vi "Get Position.vi"(8 "error in (no error)":errorcluster, 11 "KUKA youBot gripper motor_EtherCAT in":refnum<class "NI_Robotics_KUKA youBot Gripper Motor_EtherCAT.lvclass">) -> (0 "error out":errorcluster, 2 "position (m)":dbl, 3 "KUKA youBot gripper motor_EtherCAT out":refnum<class "NI_Robotics_KUKA youBot Gripper Motor_EtherCAT.lvclass">)   [LabVIEW 2017, in "NI_Robotics_KUKA youBot Host.lvlib" / "NI_Robotics_KUKA youBot Gripper Motor_EtherCAT.lvclass"]
uses:
  <vilib>/robotics/KUKA youBot/Motor/Gripper Motor EtherCAT/NI_Robotics_KUKA youBot Gripper Motor_EtherCAT.lvclass
  <vilib>/robotics/KUKA youBot/Motor/Gripper Motor EtherCAT/NI_Robotics_KUKA youBot Gripper Motor_EtherCAT.lvclass/NI_Robotics_KUKA youBot Gripper Motor_EtherCAT.ctl
  <vilib>/robotics/KUKA youBot/EtherCAT/EtherCAT Command.ctl
  <vilib>/robotics/KUKA youBot/EtherCAT/CmdCtrls/Param Cmd.ctl
  <vilib>/robotics/KUKA youBot/NI_Robotics_KUKA youBot Host.lvlib
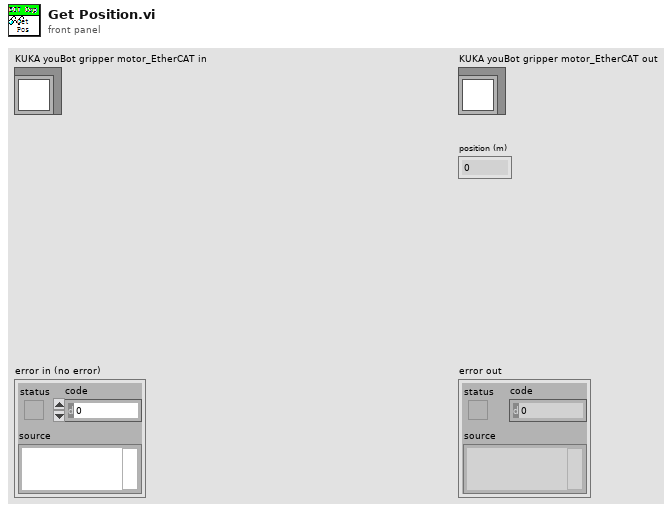
[diagram p1: front panel]
types:
  T1 = typedef "NI_Robotics_KUKA youBot Host.lvlib/EtherCAT Command.ctl" = cluster{"Module":u8, "Cmd":T2, "Type":u8, "Bank":u8, "Val":u32}
  T2 = typedef "NI_Robotics_KUKA youBot Host.lvlib/Param Cmd.ctl" = u8
  T3 = typedef "NI_Robotics_KUKA youBot Host.lvlib/Mater Handler.ctl" = i32
  T4 = typedef "NI_Robotics_KUKA youBot Host.lvlib/EtherCAT Reply.ctl" = cluster{"replyAddr":u8, "moduleAddr":u8, "status":u8, "Cmd":u8, "Val":i32}
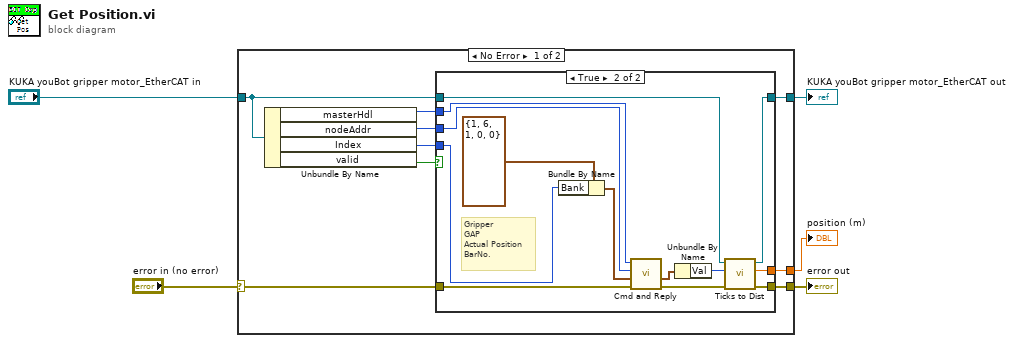
[diagram p0: block diagram]
diagram:
  n1 = case shown="No Error" "error in (no error)" {
    selector: "error in (no error)" -> [w13 w30]
    tunnel: "KUKA youBot gripper motor_EtherCAT in" -> [w9 w31]
    tunnel: [w8 _] -> w3
    tunnel: [w7 w30] -> w2
    tunnel: [w6 w31] -> w1
    frame No Error {
      n2 = Unbundle By Name(w9) -> ("masterHdl"=w11:T3, "nodeAddr"=w10:u16, "Index"=w12:i32, "valid"=w14:bool)
      n3 = case shown="True" w14 {
        tunnel: w13 -> [w15 w29]
        tunnel: w12 -> [_ w27]
        tunnel: w11 -> [_ w25]
        tunnel: w10 -> [_ w24]
        tunnel: w9 -> [w16 w20]
        tunnel: [_ w17] -> w8
        tunnel: [w15 w19] -> w7
        tunnel: [w16 w18] -> w6
        frame False {
        }
        frame True {
          # "Gripper\nGAP\nActual Position\nBarNo."
          n4 = Bundle By Name(cluster=T1 {"Module"=1, "Cmd"=6, "Type"=1, "Bank"=0, "Val"=0} ("EtherCAT Command"), "Bank"=w27) -> (w26:T1)
          n5 = call <vilib>:"Cmd and Reply.vi"("error in (no error)"=w29, "EtherCAT command"=w26, "nodeAddr in"=w24, "masterHdl in"=w25) -> ("error out"=w22:errorcluster, "EtherCAT reply"=w23:T4)  [unwired: 3 in, 3 out]
          n6 = Unbundle By Name(w23) -> ("Val"=w21:i32)
          n7 = call <vilib>:"Ticks to Dist.vi"("error in (no error)"=w22, "ticks"=w21, "KUKA youBot gripper motor_EtherCAT in"=w20) -> ("error out"=w19:errorcluster, "distance (m)"=w17:dbl, "KUKA youBot gripper motor_EtherCAT out"=w18:refnum<class "NI_Robotics_KUKA youBot Gripper Motor_EtherCAT.lvclass">)  [unwired: 6 in]
        }
      }
    }
    frame Error {
    }
  }
  "error out" <- w2
  "KUKA youBot gripper motor_EtherCAT out" <- w1
  "position (m)" <- w3
